vi "Engine In - Sensor - EGR Differential Pressure.vi"(10 "Loop Freq (Hz)":sgl, 11 "EGR Differential Pressure [V]":sgl) -> (3 "EGR Differential Pressure [kPa]":sgl)   [LabVIEW 2015, in "ECS-RT.lvlib"]
uses:
  ECS-RT.lvlib
  <vilib>/ptbypt/NI_PtbyPt.lvlib
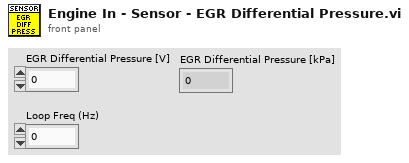
[diagram p1: front panel]
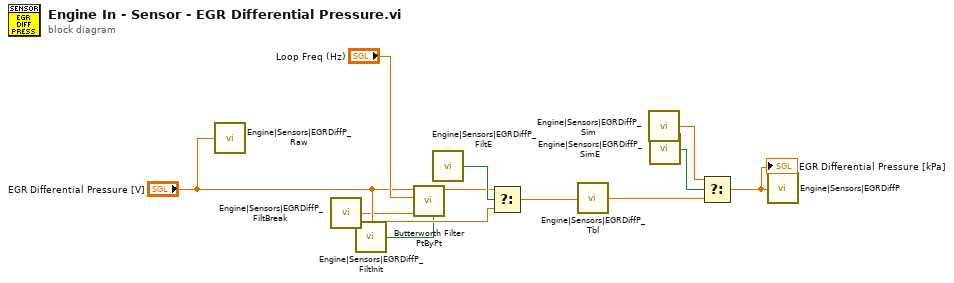
[diagram p0: block diagram]
diagram:
  n1 = call "Engine|Sensors|EGRDiffP_Raw"("Value"="EGR Differential Pressure [V]") -> ()
  n2 = call "Engine|Sensors|EGRDiffP_FiltBreak"() -> ("Value"=w6:sgl)
  n3 = call "Engine|Sensors|EGRDiffP_FiltInit"() -> ("Value"=w3:bool)
  n4 = call <vilib>:"Butterworth Filter PtByPt.vi"("initialize"=w3, "low cutoff freq: fl"=w6, "sampling freq: fs"="Loop Freq (Hz)", "x"="EGR Differential Pressure [V]") -> ("Filtered x"=w4:dbl)  [unwired: 5 in, 1 out]
  n5 = call "Engine|Sensors|EGRDiffP_FiltE"() -> ("Value"=w7:bool)
  n6 = Select(t=w4, s=w7, f="EGR Differential Pressure [V]") -> (s? t:f=w5:dbl)
  n7 = call "Engine|Sensors|EGRDiffP_Tbl"("X Index"=w5) -> ("Y"=w8:sgl)
  n8 = call "Engine|Sensors|EGRDiffP_Sim"() -> ("Value"=w2:sgl)
  n9 = call "Engine|Sensors|EGRDiffP_SimE"() -> ("Value"=w9:bool)
  n10 = Select(t=w2, s=w9, f=w8) -> (s? t:f=w1:sgl)
  "EGR Differential Pressure [kPa]" <- w1
  n11 = call "Engine|Sensors|EGRDiffP"("Value"=w1) -> ()
